vi "BRig_Host_dataRunState_dataPlot_timeout.vi"() -> (2 "output_idx_dataPlot_timeout":i32)   [LabVIEW 2014]
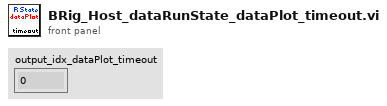
[diagram p1: front panel]
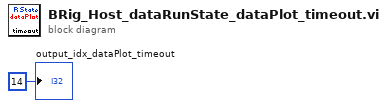
[diagram p0: block diagram]
diagram:
  "output_idx_dataPlot_timeout" <- 14 ("output_idx_dataTS")
